vi "XML Command.vi"(11 "String":string="<?xml version=\"1.0\" encoding=\"UTF-8\"?>\n<CRCLCommandInstance\n xmlns:xsi=\"http://www.w3.org/2001/XMLSchema-instance\"\n xsi:noNamespaceSchematicLocation=\"../xmlSchemas/CRCLCommandInstance.xsd\">\n  <CRCLCommand xsi:type=\"MoveToType\" >\n    <CommandID>2</CommandID>\n    <MoveStraight>false</MoveStraight>\n    <Pose>\n     <Point>\n       <X>2.5</X> <Y>1</Y> <Z>1</Z>\n     </Point>\n     <XAxis>\n       <I>1</I> <J>0</J> <K>0</K>\n     </XAxis>\n     <ZAxis>\n       <I>0</I> <J>0</J> <K>-1</K>\n     </ZAxis>\n    </Pose>\n    <NumPositions>1</NumPositions>\n  </CRCLCommand>\n</CRCLCommandInstance>\n ") -> (1 "Parameters":string, 3 "Command":string, 4 "CommandID":i32)   [LabVIEW 2013]
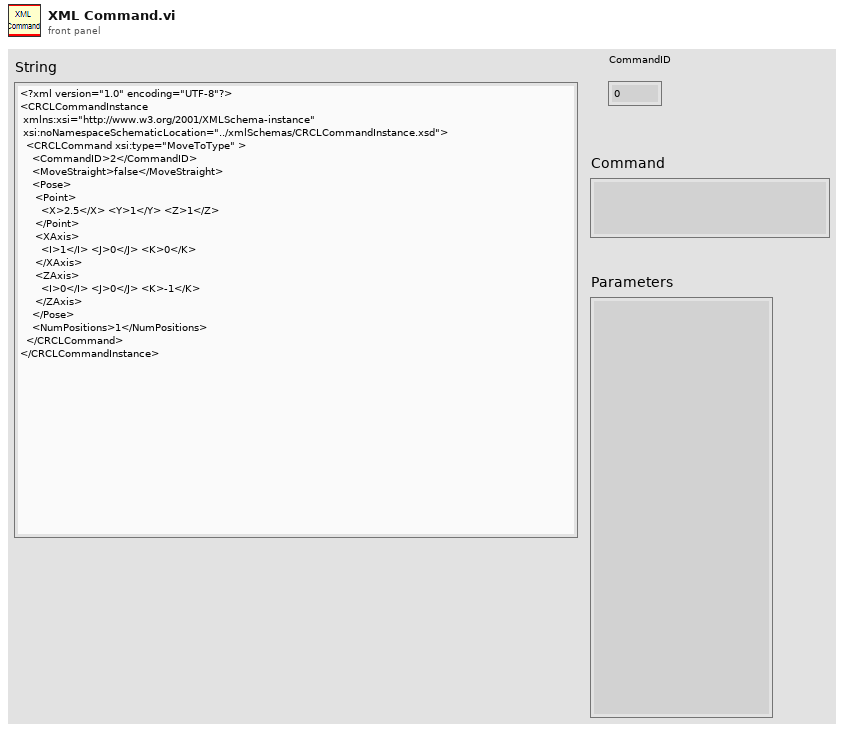
[diagram p1: front panel]
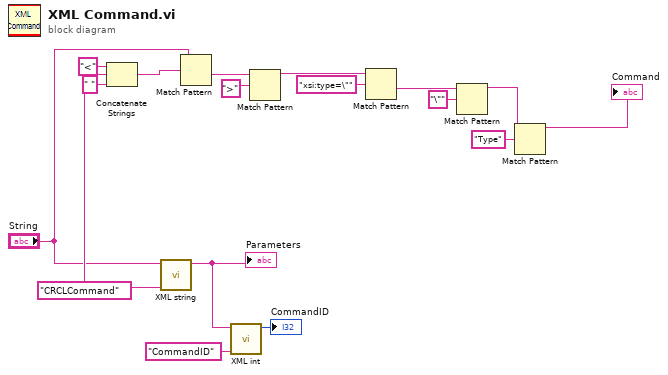
[diagram p0: block diagram]
diagram:
  w11 = "CRCLCommand" ("regular expression")
  n1 = Concatenate Strings("<" ("string"), w11, " " ("string")) -> (w12:string)
  n2 = call "XML string.vi"("tag"=w11, "String"="String") -> ("string"=w17:string)  [unwired: 8 in, 1 out]
  "Parameters" <- w17
  n3 = Match Pattern(string="String", regular expression=w12) -> (after substring=w14:string)  [unwired: 1 in, 3 out]
  n4 = call "XML int.vi"("tag"="CommandID", "String"=w17) -> ("int"=→"CommandID":i32)  [unwired: 9 in]
  n5 = Match Pattern(string=w14, regular expression=">") -> (before substring=w8:string)  [unwired: 1 in, 3 out]
  n6 = Match Pattern(string=w8, regular expression="xsi:type=\"") -> (after substring=w6:string)  [unwired: 1 in, 3 out]
  n7 = Match Pattern(string=w6, regular expression="\"") -> (before substring=w3:string)  [unwired: 1 in, 3 out]
  n8 = Match Pattern(string=w3, regular expression="Type") -> (before substring=→"Command":string)  [unwired: 1 in, 3 out]
